vi "distibution generator.vi"(0 "samples":i32=35, 2 "mean (ns)":dbl=3421563217743244.0 format="%_15g", 11 "standard deviation (ns)":dbl=437.0, 13 "dist choice (T=flat/F=gauss)":bool) -> (8 "time cluster array out":T1[](array[typedef])=[{"day"=39, "hour"=14, "min"=26, "sec"=3, "msec"=217, "usec"=743, "nsec"=67}, {"day"=39, "hour"=14, "min"=26, "sec"=3, "msec"=217, "usec"=743, "nsec"=441}, {"day"=39, "hour"=14, "min"=26, "sec"=3, "msec"=217, "usec"=743, "nsec"=8}, {"day"=39, "hour"=14, "min"=26, "sec"=3, "msec"=217, "usec"=743, "nsec"=29}, {"day"=39, "hour"=14, "min"=26, "sec"=3, "msec"=217, "usec"=742, "nsec"=693}, {"day"=39, "hour"=14, "min"=26, "sec"=3, "msec"=217, "usec"=743, "nsec"=422}, {"day"=39, "hour"=14, "min"=26, "sec"=3, "msec"=217, "usec"=741, "nsec"=839}, {"day"=39, "hour"=14, "min"=26, "sec"=3, "msec"=217, "usec"=743, "nsec"=166}, {"day"=39, "hour"=14, "min"=26, "sec"=3, "msec"=217, "usec"=743, "nsec"=635}, {"day"=39, "hour"=14, "min"=26, "sec"=3, "msec"=217, "usec"=743, "nsec"=781}, {"day"=39, "hour"=14, "min"=26, "sec"=3, "msec"=217, "usec"=743, "nsec"=705}, {"day"=39, "hour"=14, "min"=26, "sec"=3, "msec"=217, "usec"=743, "nsec"=49}, {"day"=39, "hour"=14, "min"=26, "sec"=3, "msec"=217, "usec"=743, "nsec"=277}, {"day"=39, "hour"=14, "min"=26, "sec"=3, "msec"=217, "usec"=743, "nsec"=509}, {"day"=39, "hour"=14, "min"=26, "sec"=3, "msec"=217, "usec"=743, "nsec"=611}, {"day"=39, "hour"=14, "min"=26, "sec"=3, "msec"=217, "usec"=743, "nsec"=29}, {"day"=39, "hour"=14, "min"=26, "sec"=3, "msec"=217, "usec"=743, "nsec"=126}, {"day"=39, "hour"=14, "min"=26, "sec"=3, "msec"=217, "usec"=744, "nsec"=29}, {"day"=39, "hour"=14, "min"=26, "sec"=3, "msec"=217, "usec"=743, "nsec"=886}, {"day"=39, "hour"=14, "min"=26, "sec"=3, "msec"=217, "usec"=743, "nsec"=544}, {"day"=39, "hour"=14, "min"=26, "sec"=3, "msec"=217, "usec"=742, "nsec"=366}, {"day"=39, "hour"=14, "min"=26, "sec"=3, "msec"=217, "usec"=743, "nsec"=623}, {"day"=39, "hour"=14, "min"=26, "sec"=3, "msec"=217, "usec"=743, "nsec"=115}, {"day"=39, "hour"=14, "min"=26, "sec"=3, "msec"=217, "usec"=743, "nsec"=391}, {"day"=39, "hour"=14, "min"=26, "sec"=3, "msec"=217, "usec"=743, "nsec"=5}, {"day"=39, "hour"=14, "min"=26, "sec"=3, "msec"=217, "usec"=743, "nsec"=326}, {"day"=39, "hour"=14, "min"=26, "sec"=3, "msec"=217, "usec"=743, "nsec"=118}, {"day"=39, "hour"=14, "min"=26, "sec"=3, "msec"=217, "usec"=743, "nsec"=463}, {"day"=39, "hour"=14, "min"=26, "sec"=3, "msec"=217, "usec"=742, "nsec"=940}, {"day"=39, "hour"=14, "min"=26, "sec"=3, "msec"=217, "usec"=743, "nsec"=186}, {"day"=39, "hour"=14, "min"=26, "sec"=3, "msec"=217, "usec"=743, "nsec"=592}, {"day"=39, "hour"=14, "min"=26, "sec"=3, "msec"=217, "usec"=743, "nsec"=70}, {"day"=39, "hour"=14, "min"=26, "sec"=3, "msec"=217, "usec"=742, "nsec"=922}, {"day"=39, "hour"=14, "min"=26, "sec"=3, "msec"=217, "usec"=742, "nsec"=56}, {"day"=39, "hour"=14, "min"=26, "sec"=3, "msec"=217, "usec"=743, "nsec"=210}])   [LabVIEW 2014]
doc: "This subVI generates time cluster arrays for use in Exercise 4.\n\nPaul K Dixon\nP350\nCSUSB Physics"
uses:
  typedefs/time cluster typedef.ctl
  <vilib>/Analysis/NI_AALBase.lvlib
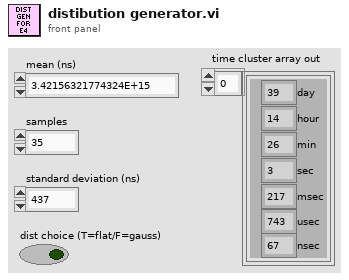
[diagram p1: front panel]
types:
  T1 = typedef "time cluster typedef.ctl" = cluster{"day":u32, "hour":u32, "min":u32, "sec":u32, "msec":u32, "usec":u32, "nsec":u32}
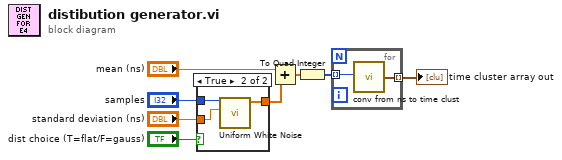
[diagram p0: block diagram]
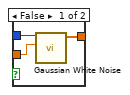
[diagram p2: hidden frame]
diagram:
  n1 = case shown="True" "dist choice (T=flat/F=gauss)" {
    tunnel: "samples" -> [w11 w14]
    tunnel: "standard deviation (ns)" -> [w10 w13]
    tunnel: [w9 w12] -> w7
    frame False {
      n2 = call <vilib>:"Gaussian White Noise.vi"("standard deviation"=w10, "samples"=w11) -> ("Gaussian noise pattern"=w9:dbl[])  [unwired: 8 in, 1 out]
    }
    frame True {
      n3 = call <vilib>:"Uniform White Noise.vi"("amplitude"=w13, "samples"=w14) -> ("uniform white noise"=w12:dbl[])  [unwired: 8 in, 1 out]
    }
  }
  n4 = Add(x="mean (ns)", y=w7) -> (x+y=w3:dbl[])
  n5 = To Quad Integer(1:w3) -> (0:w2:i64[])
  n6 = for {
    tunnel: w2 -> [w16] mode=indexing
    tunnel: [w15] -> w4 mode=indexing
    n7 = call "conv from ns to time clust.vi"("time (nsec)"=w16) -> ("time cluster"=w15:T1)  [unwired: 13 in, 1 out]
  }
  "time cluster array out" <- w4
